vi "TeamMove.vi"(8 "error in (no error)":errorcluster, 11 "TeamEffort in":refnum<class "TeamEffort.lvclass">) -> (0 "error out":errorcluster, 1 "Direction":T1, 2 "Action":T2, 3 "TeamEffort out":refnum<class "TeamEffort.lvclass">, 4 "Replicated":refnum<class "Square.lvclass">)   [LabVIEW 2014, in "TeamEffort.lvclass"]
uses:
  TeamEffort.lvclass
  SquareBattle Arena/Action Enum.ctl
  SquareBattle Arena/Direction Enum.ctl
  Square.lvclass
  SquareBattle Arena/SquareBattle Arena.lvclass
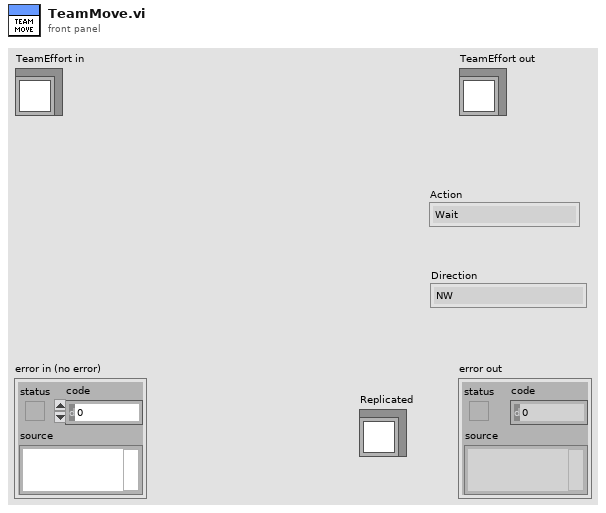
[diagram p1: front panel]
types:
  T1 = typedef "SquareBattle Arena.lvlib/SquareBattle Arena.lvclass/Direction Enum.ctl" = enum16{"NW", "N", "NE", "E", "SE", "S", "SW", "W"}
  T2 = typedef "SquareBattle Arena.lvlib/SquareBattle Arena.lvclass/Action Enum.ctl" = enum16{"Wait", "Move", "Attack", "Replicate"}
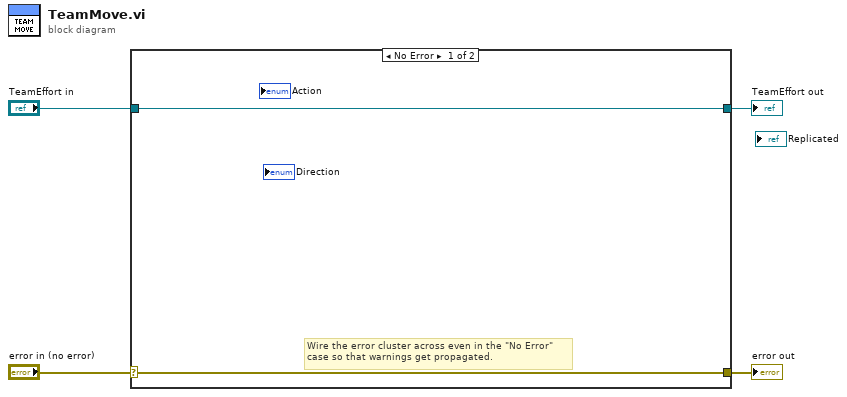
[diagram p0: block diagram]
diagram:
  n1 = case shown="No Error" "error in (no error)" {
    selector: "error in (no error)" -> [w5 w8]
    tunnel: [w5 w8] -> w3
    tunnel: [w6 w7] -> w1
    tunnel: "TeamEffort in" -> [w6 w7]
    frame No Error {
      # "Wire the error cluster across even in the \"No Error\"\ncase so that warnings get propagated."
    }
    frame Error {
    }
  }
  "error out" <- w3
  "TeamEffort out" <- w1
